vi "Calculate Efficiency.vi"(8 "load current measurements":dbl[](array[numeric]), 9 "load voltage measurements":dbl[](array[numeric]), 10 "source current measurements":dbl[](array[numeric]), 11 "source voltage measurements":dbl[](array[numeric])) -> (3 "Efficiency(%)":dbl[](array[numeric]))   [LabVIEW 2021, in "Efficiency And Load Regulation with Pin Map.lvlib"]
uses:
  Efficiency And Load Regulation with Pin Map.lvlib
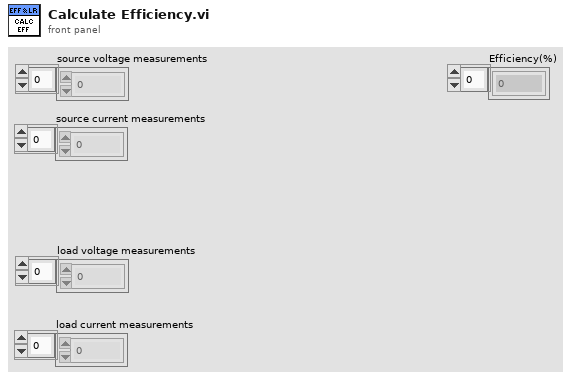
[diagram p1: front panel]
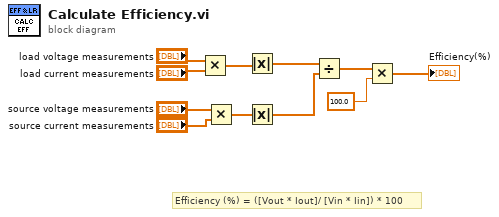
[diagram p0: block diagram]
diagram:
  # "Efficiency (%) = ([Vout * Iout]/ [Vin * Iin]) * 100"
  n1 = Multiply(x="load voltage measurements", y="load current measurements") -> (x*y=w6:dbl[])
  n2 = Multiply(x="source voltage measurements", y="source current measurements") -> (x*y=w5:dbl[])
  n3 = Absolute Value(x=w6) -> (abs(x)=w11:dbl[])
  n4 = Absolute Value(x=w5) -> (abs(x)=w10:dbl[])
  n5 = Divide(x=w11, y=w10) -> (x/y=w9:dbl[])
  n6 = Multiply(x=w9, y=100.0) -> (x*y=→"Efficiency(%)":dbl[])
